vi "createNewArrayObject.vi"(8 "error in (no error)":errorcluster, 10 "arrayRef":refnum<vi>, 11 "LongLong in":refnum<class "LongLong.lvclass">) -> (0 "error out":errorcluster, 3 "LongLong out":refnum<class "LongLong.lvclass">)   [LabVIEW 2016, in "LongLong.lvclass"]
uses:
  LongLong.lvclass
  home/andres/ts_sallabview/SALTypeGenerator/Elements/Numeric/Numeric.lvclass
  <vilib>/numeric/LVNumericRepresentation.ctl
  Numeric/Numeric.lvclass/Numeric.ctl
  Signed/Signed.lvclass
  Numeric/Numeric.lvclass
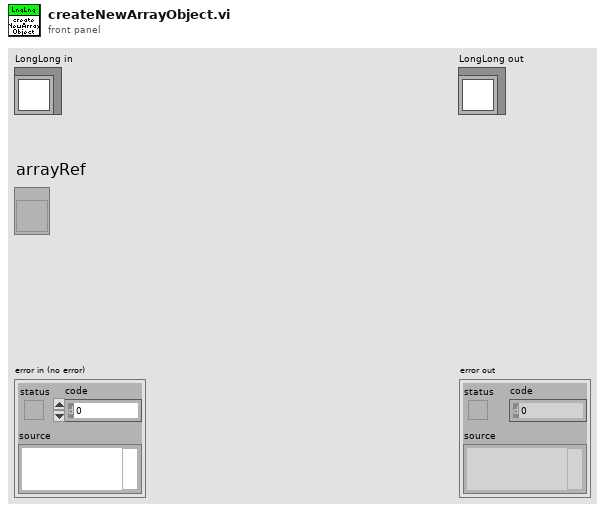
[diagram p1: front panel]
types:
  T1 = typedef "LVNumericRepresentation.ctl" = enum32{"Extended Precision", "Double Precision", "Single Precision", "Long", "Word", "Byte", "Unsigned Long", "Unsigned Word", "Unsigned Byte", "Complex Extended", "Complex Double", "Complex Single", "Quad", "Unsigned Quad", "Fixed-Point"}
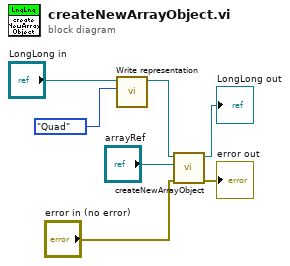
[diagram p0: block diagram]
diagram:
  n1 = call "Write representation.vi"("Numeric Representation"=LVNumericRepresentation."Quad", "Numeric in"="LongLong in") -> ("Numeric out"=w2:refnum<class "LongLong.lvclass">)  [unwired: 9 in]
  n2 = call-parent "createNewArrayObject.vi"("error in (no error)"="error in (no error)", "arrayRef"="arrayRef", "Numeric in"=w2) -> ("error out"=→"error out":errorcluster, "Numeric out"=→"LongLong out":refnum<class "LongLong.lvclass">)  [unwired: 7 in]
